vi "Turn to angle computation.vi"(8 "Current Angle":dbl(slide) scale=-1000.0..1000.0, 11 "Angle To Get":dbl(slide) scale=-5000.0..5000.0) -> (1 "New Angle to get":dbl(slide) scale=-1000.0..1000.0)   [LabVIEW 2019]
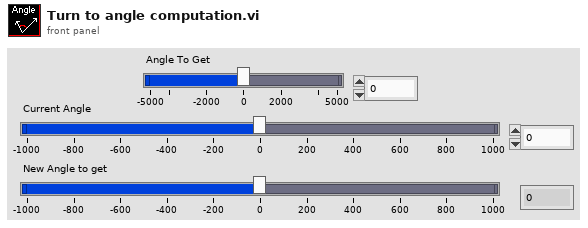
[diagram p1: front panel]
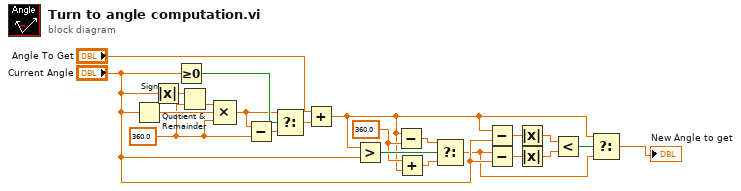
[diagram p0: block diagram]
diagram:
  w13 = 360.0 ("value")
  w1 = 360.0 ("value")
  n1 = Sign(1:"Current Angle") -> (0:w20:dbl)
  n2 = Absolute Value(x="Current Angle") -> (abs(x)=w22:dbl)
  n3 = Greater Or Equal To 0?(x="Current Angle") -> (x >= 0?=w18:bool)
  n4 = Quotient & Remainder(x=w22, y=w1) -> (floor(x/y)=w21:dbl)  [unwired: 1 out]
  n5 = Compound Arithmetic op=MULTIPLY(w21, w20, w1) -> (w16:dbl)
  n6 = Subtract(x=w16, y=w1) -> (x-y=w17:dbl)
  n7 = Select(t=w16, s=w18, f=w17) -> (s? t:f=w15:dbl)
  n8 = Add(x="Angle To Get", y=w15) -> (x+y=w4:dbl)
  n9 = Greater?(x=w4, y="Current Angle") -> (0:w14:bool)
  n10 = Subtract(x=w4, y=w13) -> (x-y=w12:dbl)
  n11 = Add(x=w13, y=w4) -> (x+y=w11:dbl)
  n12 = Select(t=w12, s=w14, f=w11) -> (s? t:f=w3:dbl)
  n13 = Subtract(x=w4, y="Current Angle") -> (x-y=w9:dbl)
  n14 = Subtract(x=w3, y="Current Angle") -> (x-y=w8:dbl)
  n15 = Absolute Value(x=w9) -> (abs(x)=w7:dbl)
  n16 = Absolute Value(x=w8) -> (abs(x)=w6:dbl)
  n17 = Less?(x=w7, y=w6) -> (x < y?=w5:bool)
  n18 = Select(t=w4, s=w5, f=w3) -> (s? t:f=→"New Angle to get":dbl)
